vi "votalge inandout.vi"() -> ()   [LabVIEW 8.6]
uses:
  <vilib>/DAQmx/write.llb/DAQmx Write (Analog DBL 1Chan 1Samp).vi
  <vilib>/DAQmx/create/channels.llb/DAQmx Create Channel (AO-Voltage-Basic).vi
panel:
  out "Numeric":dbl
  in  "Voltage in":dbl format="%0.2f"
  out "Hall Proobe":dbl
  in  "stop":bool
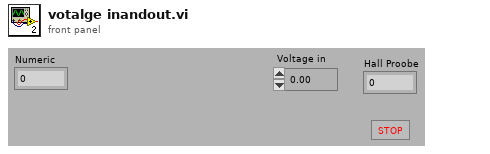
[diagram p1: front panel]
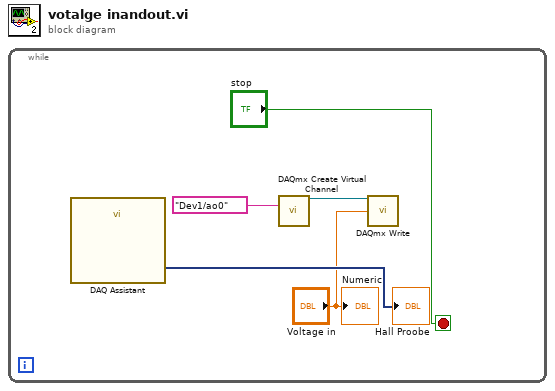
[diagram p0: block diagram]
diagram:
  n1 = while {
    stop <- "stop" stop-if-true
    n2 = call "DAQ Assistant"() -> ("data"=→"Hall Proobe":dynamicdata)  [unwired: 17 in, 2 out]
    n3 = call-poly <vilib>:"DAQmx Create Virtual Channel.vi"("physical channels"=tag "Dev1/ao0") -> ("task out"=w1:refnum<k21>)  [unwired: 13 in, 1 out]
    n4 = call-poly <vilib>:"DAQmx Write.vi"("task/channels in"=w1, "data"="Voltage in") -> ()  [unwired: 11 in, 3 out]
    "Numeric" <- "Voltage in"
  }
